vi "test1_160524.vi"() -> ()   [LabVIEW 2015]
uses:
  <vilib>/NXT/Block Support/NXT_InputPort.ctl
  <vilib>/NXT/Block Support/NXT_OutputPort.ctl
  <vilib>/NXT/Dual Mode Library/Sensors/Light_On.vi
  <vilib>/NXT/Dual Mode Library/Sensors/Sonar_cm.vi
  <vilib>/NXT/NXTIO Xnodes/NXTIONodeSubVIs/NXTMoveMotors.vi
  <vilib>/NXT/Dual Mode Library/Waits/Wait_Num.vi
  <vilib>/NXT/Subs/LVHSConnector.ctl
  <vilib>/NXT/NXTIO Xnodes/AddressXNode/NXTIOAddress.xnode
  <vilib>/NXT/NXTIO Xnodes/NXTIOXNode/NXTIO.xnode
  <vilib>/NXT/LegoClasses/BrickReference/BrickReference.lvclass
panel:
  in  "turn lefttC 2":i8=75
  in  "turn lefttB 2":i8=75
  in  "Go-ahead":i8=75
  out "check destance":i16(slide) scale=0.0..100.0
  in  "turn rightC":i8=75
  in  "turn rightB":i8=75
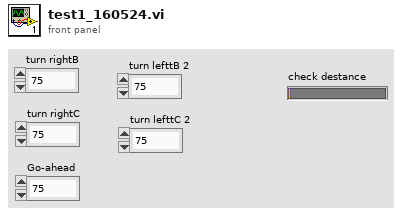
[diagram p1: front panel]
types:
  T1 = typedef "NXT_OutputPort.ctl" = u8
  T2 = typedef "NXT_InputPort.ctl" = u32
  T3 = typedef "LVHSConnector.ctl" = refnum<class "BrickReference.lvclass">
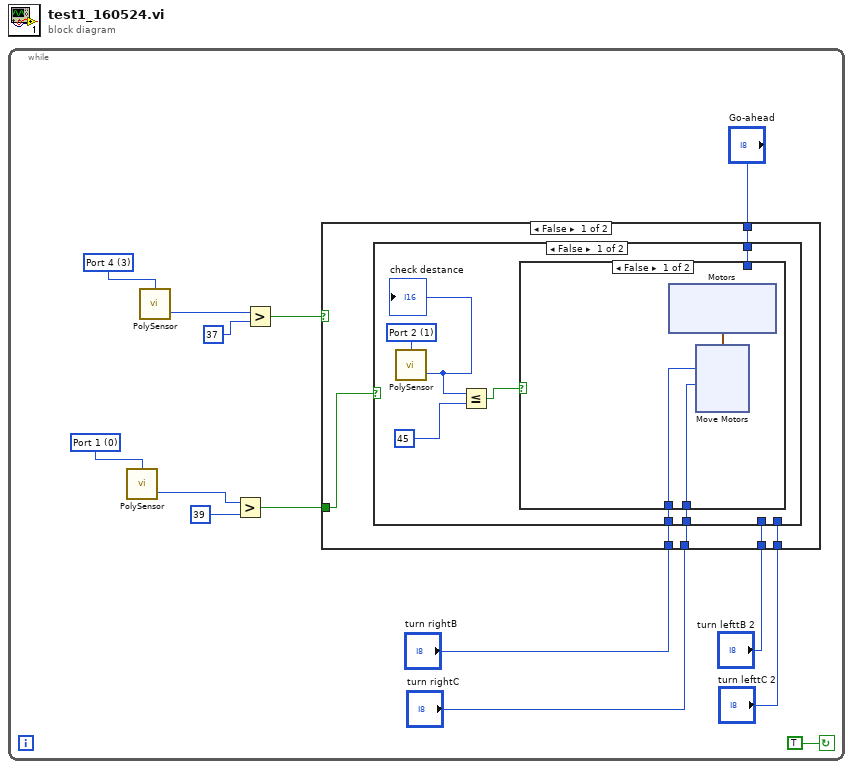
[diagram p0: block diagram]
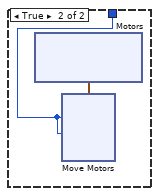
[diagram p2: hidden frame]
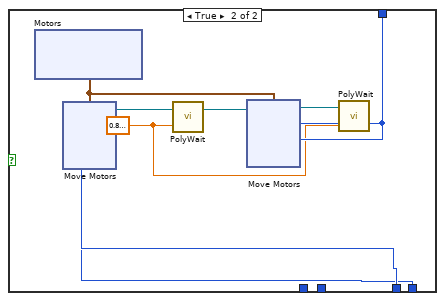
[diagram p3: hidden frame]
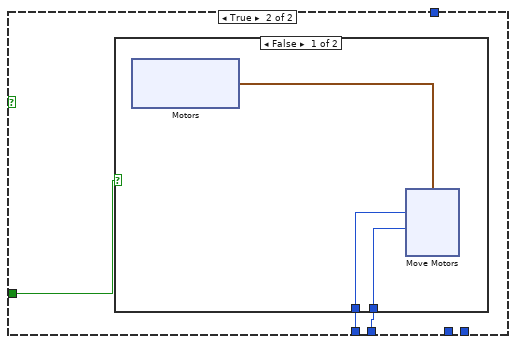
[diagram p4: hidden frame]
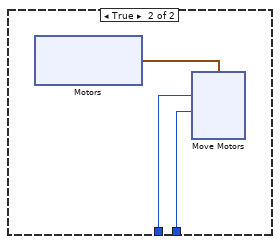
[diagram p5: hidden frame]
diagram:
  n1 = while {
    stop <- TRUE continue-if-true
    w10 = T2 3 items=["Port 1", "Port 2", "Port 3", "Port 4"] ("Port (Port 3)")
    w9 = T2 0 items=["Port 1", "Port 2", "Port 3", "Port 4"] ("Port (Port 3)")
    n2 = call-poly <vilib>:"PolySensor.vi"("Port (Port 3)"=w9) -> ("Scaled Value"=w11:i16)  [unwired: 2 in, 1 out]
    n3 = call-poly <vilib>:"PolySensor.vi"("Port (Port 3)"=w10) -> ("Scaled Value"=w13:i16)  [unwired: 2 in, 1 out]
    n4 = Greater?(x=w11, y=i16 39) -> (0:w7:bool)
    n5 = Greater?(x=w13, y=i16 37) -> (0:w8:bool)
    n6 = case shown="False" w8 {
      tunnel: w7 -> [w20 w78]
      tunnel: "turn rightB" -> [w19 w77]
      tunnel: "turn rightC" -> [w18 w76]
      tunnel: "Go-ahead" -> [w17 _]
      tunnel: "turn lefttB 2" -> [w16 _]
      tunnel: "turn lefttC 2" -> [w15 _]
      frame False {
        n7 = case shown="False" w20 {
          tunnel: w19 -> [w27 _]
          tunnel: w18 -> [w26 _]
          tunnel: w17 -> [w21 w54]
          tunnel: w16 -> [_ w58]
          tunnel: w15 -> [_ w57]
          frame False {
            w24 = T2 1 items=["Port 1", "Port 2", "Port 3", "Port 4"] ("Port (Port 4)")
            n8 = call-poly <vilib>:"PolySensor.vi"("Port (Port 4)"=w24) -> ("Distance (cm)"=w25:i16)  [unwired: 2 in, 1 out]
            "check destance" <- w25
            n9 = Less Or Equal?(x=w25, y=i16 45) -> (x <= y?=w22:bool)
            n10 = case shown="False" w22 {
              tunnel: w27 -> [w29 _]
              tunnel: w26 -> [w28 _]
              tunnel: w21 -> [_ w40]
              frame False {
                n11 = xnode "Motors"() -> ("Motor"=w30:cluster{"Port":T1, "Port":T1})
                n12 = xnode "Move Motors"("Power/Speed 2"=w28, "Power/Speed 1"=w29, "Motors"=w30) -> ()  [unwired: 1 in, 1 out]
              }
              frame True {
                n13 = xnode "Motors"() -> ("Motor"=w41:cluster{"Port":T1, "Port":T1})
                n14 = xnode "Move Motors"("Power/Speed 2"=w40, "Power/Speed 1"=w40, "Motors"=w41) -> ()  [unwired: 1 in, 1 out]
              }
            }
          }
          frame True {
            w51 = sgl 0.8 ("Time (1 sec)")
            n15 = xnode "Motors"() -> ("Motor"=w55:cluster{"Port":T1, "Port":T1})
            n16 = xnode "Move Motors"("Power/Speed 2"=w57, "Power/Speed 1"=w58, "Motors"=w55) -> ("NXT/EV3"=w56:T3)  [unwired: 1 in]
            n17 = call-poly <vilib>:"PolyWait.vi"("Time (1 sec)"=w51, "NXT/EV3"=w56) -> ("NXT/EV3"=w53:T3)  [unwired: 2 in]
            n18 = xnode "Move Motors"("Power/Speed 2"=w54, "Power/Speed 1"=w54, "Motors"=w55, "NXT/EV3"=w53) -> ("NXT/EV3"=w52:T3)
            n19 = call-poly <vilib>:"PolyWait.vi"("Time (1 sec)"=w51, "NXT/EV3"=w52) -> ()  [unwired: 2 in, 1 out]
          }
        }
      }
      frame True {
        n20 = case shown="False" w78 {
          tunnel: w77 -> [w79 w92]
          tunnel: w76 -> [w80 w91]
          frame False {
            n21 = xnode "Motors"() -> ("Motor"=w81:cluster{"Port":T1, "Port":T1})
            n22 = xnode "Move Motors"("Power/Speed 2"=w80, "Power/Speed 1"=w79, "Motors"=w81) -> ()  [unwired: 1 in, 1 out]
          }
          frame True {
            n23 = xnode "Motors"() -> ("Motor"=w93:cluster{"Port":T1, "Port":T1})
            n24 = xnode "Move Motors"("Power/Speed 2"=w91, "Power/Speed 1"=w92, "Motors"=w93) -> ()  [unwired: 1 in, 1 out]
          }
        }
      }
    }
  }
